vi "LVClass_HasoEngine Get Spot Tracker Enabled.vi"(0 "HasoEngine in":refnum<class "HasoEngine.lvclass">, 11 "error in (no error)":errorcluster) -> (4 "HasoEngine out":refnum<class "HasoEngine.lvclass">, 6 "SpotTrackerEnable":bool, 15 "error out":errorcluster)   [LabVIEW 2020, in "HasoEngine.lvclass"]
doc: "Spots detection algorithm type setter.\n\n--------------------------------------------------------------------------------\n\n<B>HasoEngineIn </B> : HasoEngine object.\n<B>HasoEngineOut </B> : HasoEngine object.\n<B>algo_type </B> : Spot tracker algorithm type : standard (0) or fast (1).\n<B>ErrorIn </B> : Error\n<B>ErrorOut </B> : Error\n\n--------------------------------------------------------------------------------"
uses:
  HasoEngine.lvclass
  HasoEngine.lvclass/HasoEngine.ctl
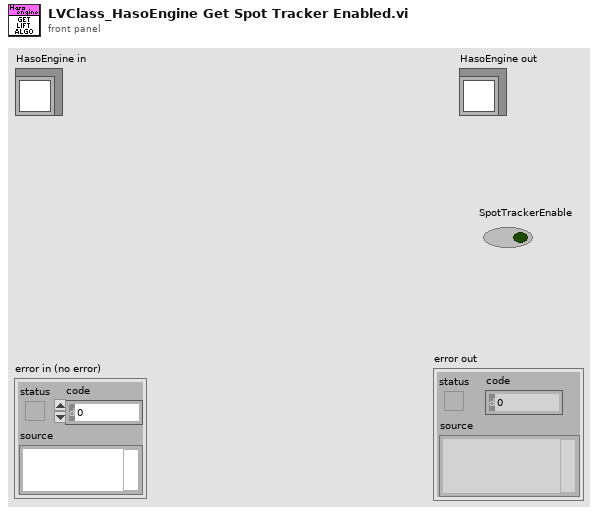
[diagram p1: front panel]
types:
  T1 = typedef "ClassID.ctl" = i64
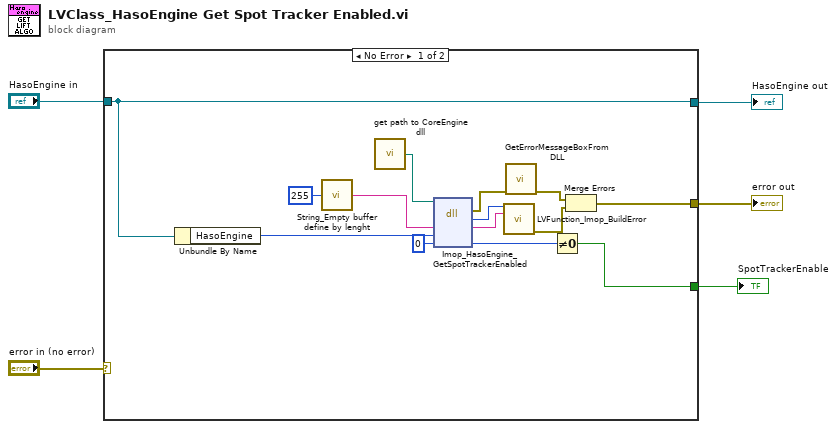
[diagram p0: block diagram]
diagram:
  n1 = case shown="No Error" "error in (no error)" {
    selector: "error in (no error)" -> [_ w20]
    tunnel: "HasoEngine in" -> [w14 w21]
    tunnel: [w14 w21] -> w2
    tunnel: [w9 w20] -> w3
    tunnel: [w6 _] -> w1
    frame No Error {
      n2 = Unbundle By Name(w14) -> ("HasoEngine"=w13:T1)
      n3 = call "String_Empty buffer define by lenght.vi"("Lenght (255)"=255) -> ("Empty buffer"=w17:string)
      n4 = call "get path to CoreEngine dll.vi"() -> ("path to wavekit library"=w16:path)  [unwired: 14 in, 1 out]
      n5 = dll-call lib="D:/soft/HASO_v3/SVN_trunk/ImOpCoreEngine4_LV2011/DLLs/c_interface_vc100.dll" fn="Imop_HasoEngine_GetSpotTrackerEnabled"(path in=w16, "message"=w17, "hasoEngine"=w13, "enable_spot_tracker"=u8 0) -> (error out=w15:errorcluster, "return type"=w18:i32, "message"=w19:string, "enable_spot_tracker"=w7:u8)  [unwired: 3 in, 1 out]
      n6 = call "LVFunction_Imop_BuildError.vi"("code"=w18, "String to Prepend to source (\"\")"=w19) -> ("error out"=w10:errorcluster)  [unwired: 13 in]
      n7 = call "GetErrorMessageBoxFromDLL.vi"("error IN"=w15) -> ("error OUT"=w11:errorcluster)  [unwired: 10 in]
      n8 = Not Equal To 0?(x=w7) -> (x != 0?=w6:bool)
      n9 = Merge Errors(w11, w10) -> (w9:errorcluster)
    }
    frame Error {
    }
  }
  "error out" <- w3
  "HasoEngine out" <- w2
  "SpotTrackerEnable" <- w1
